vi "Power Spectrum.vi"() -> ()   [LabVIEW 2015]
uses:
  <vilib>/Analysis/2dsp.llb/Real FFT.vi
  <vilib>/Analysis/NI_AALPro.lvlib
panel:
  in  "stop":bool
  out "Power Spectrum":cluster{"Elevation":sgl, dbl, dbl[]}(graph)
  in  "BW":i32
  in  "Active Antenna":string(combo)="RX1"
  in  "Gain [dB]":dbl=20.0 format="%#.6p"
  in  "Carrier\nFrequency [Hz]":dbl=90500000.0 format="%#.6p"
  in  "IQ Sampling\nRate [S/sec]":dbl=200000.0 format="%#.6p"
  in  "device name":refnum<k15>="192.168.10.2"
  # "USRP Configuration"
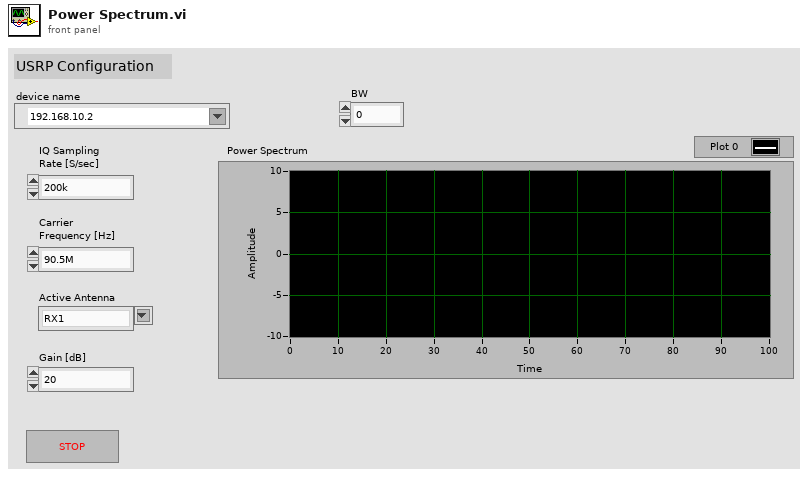
[diagram p1: front panel]
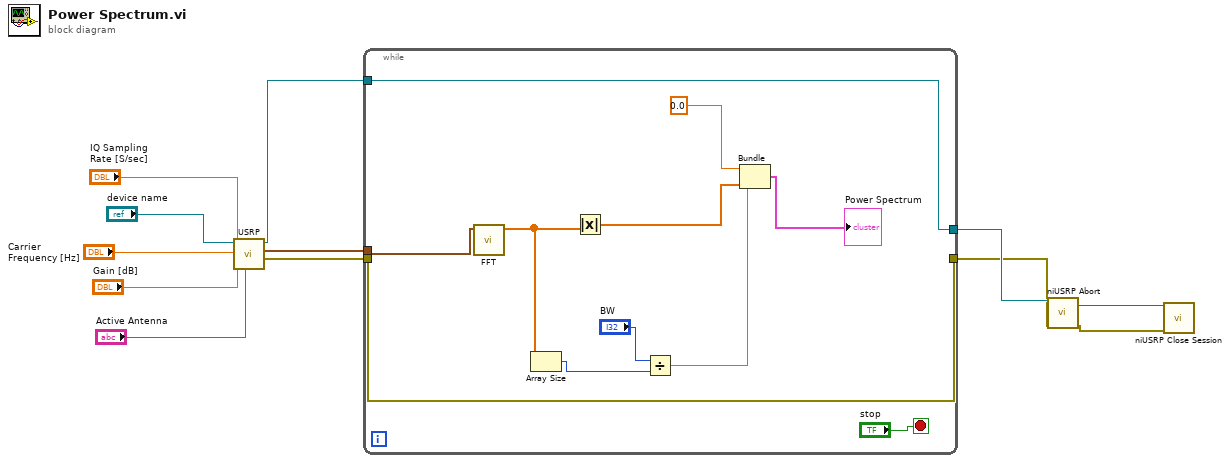
[diagram p0: block diagram]
diagram:
  n1 = call "USRP.vi"("Active Antenna"="Active Antenna", "Gain [dB]"="Gain [dB]", "Carrier\nFrequency [Hz]"="Carrier\nFrequency [Hz]", "IQ Sampling\nRate [S/sec]"="IQ Sampling\nRate [S/sec]", "device name"="device name") -> ("error out"=w2:errorcluster, "data"=w3:waveform(cdb), "session handle out"=w4:refnum<k15>)  [unwired: 4 in]
  n2 = while {
    tunnel: [w16] -> w5
    tunnel: w4 -> [w16]
    tunnel: [w15] -> _
    tunnel: w3 -> [w15]
    tunnel: w2 -> [w14]
    tunnel: [w14] -> w1
    stop <- "stop" stop-if-true
    n3 = call-poly <vilib>:"FFT.vi"("X"=w15) -> ("FFT {X}"=w17:cdb[])  [unwired: 9 in, 1 out]
    n4 = Array Size(array=w17) -> (size(s)=w18:i32)
    n5 = Absolute Value(x=w17) -> (abs(x)=w20:dbl[])
    n6 = Divide(x="BW", y=w18) -> (x/y=w21:dbl)
    n7 = Bundle("Elevation"=sgl 0.0, w21, w20) -> (→"Power Spectrum":cluster{"Elevation":sgl, dbl, dbl[]})  [unwired: 1 in]
  }
  n8 = call <instrlib>:"niUSRP Abort.vi"("session handle"=w5, "error in (no error)"=w1) -> ("session handle out"=w7:refnum<k15>, "error out"=w6:errorcluster)  [unwired: 12 in]
  n9 = call <instrlib>:"niUSRP Close Session.vi"("session handle"=w7, "error in (no error)"=w6) -> ()  [unwired: 13 in, 1 out]
